vi "Recursive Find Config File.vi"(8 "error in":errorcluster, 10 "Path":path, 11 "Configuration in":refnum<class "Configuration.lvclass">) -> (0 "error out":errorcluster, 2 "File Path":path, 3 "Configuration out":refnum<class "Configuration.lvclass">)   [LabVIEW 2018, in "Configuration.lvlib" / "Configuration.lvclass"]
doc: "This is a recursive file searcher. \n\nIt starts at an input path, moves up one directory and searches for config.ini\n\nTypical practice is to pass in the application path which will root the search in the projoct folders looking in higher level folders."
uses:
  Configuration.lvclass
  Configuration.lvclass/Configuration.ctl
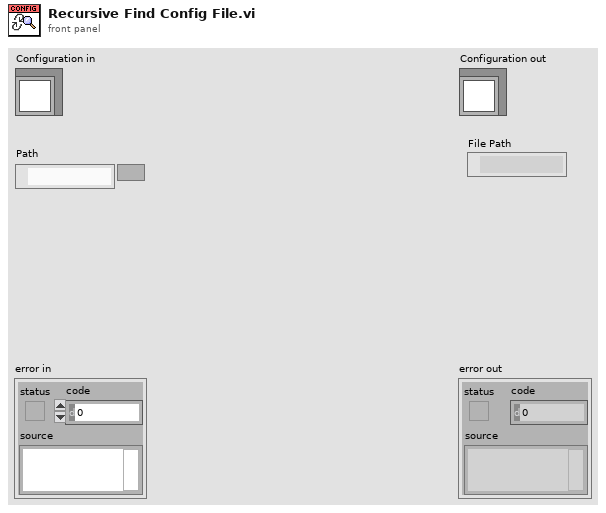
[diagram p1: front panel]
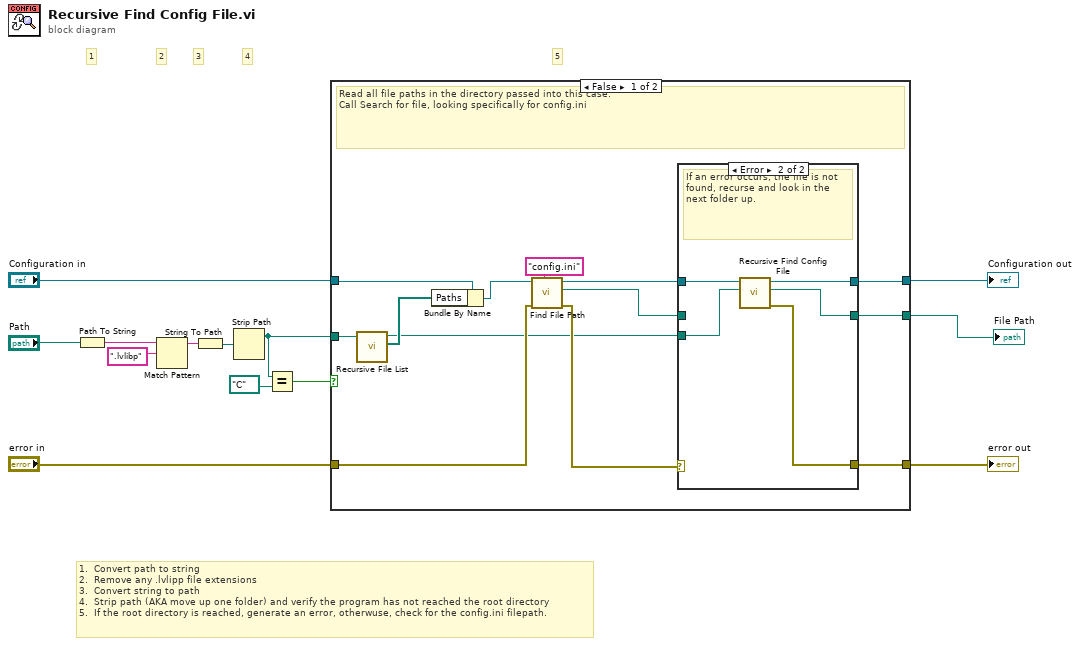
[diagram p0: block diagram]
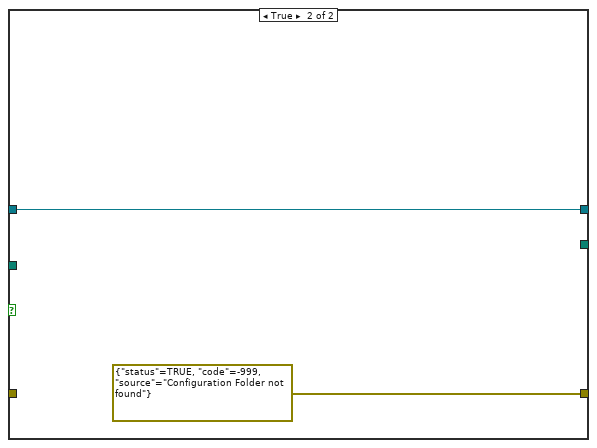
[diagram p3: hidden frame]
diagram:
  # "1.  Convert path to string\n2.  Remove any .lvlipp file extensions\n3.  Convert string to path\n4.  Strip path (AKA move up one folder) and verify the program has not reached the root directory\n5.  If the root directory is reached, generate an error, otherwuse, check for the config.ini filepath."
  # "5"
  # "4"
  # "3"
  # "2"
  # "1"
  n1 = Path To String(path="Path") -> (string=w12:string)
  n2 = Match Pattern(string=w12, regular expression=".lvlibp") -> (before substring=w10:string)  [unwired: 1 in, 3 out]
  n3 = String To Path(string=w10) -> (path=w9:path)
  n4 = Strip Path(path=w9) -> (stripped path=w6:path)  [unwired: 1 out]
  n5 = Equal?(x=w6, y=path "C:/" ("stripped path")) -> (x = y?=w7:bool)
  n6 = case shown="False" w7 {
    tunnel: w6 -> [w23 _]
    tunnel: "Configuration in" -> [w26 w36]
    tunnel: [w16 w36] -> w4
    tunnel: "error in" -> [w24 _]
    tunnel: [w15 errorcluster {"status"=TRUE, "code"=-999, "source"="Configuration Folder not found"} ("error in")] -> w2
    tunnel: [w18 _] -> w1
    frame False {
      # "Read all file paths in the directory passed into this case.\nCall Search for file, looking specifically for config.ini"
      n7 = call <vilib>:"Recursive File List.vi"("Folder Path"=w23) -> ("All Files in Dir"=w21:path[], "dup Folder Path"=w14:path)  [unwired: 6 in, 3 out]
      n8 = Bundle By Name(cluster=w26, "Paths"=w21) -> (w22:refnum<class "Configuration.lvclass">)
      n9 = call "Find File Path.vi"("error in"=w24, "Filename"="config.ini", "Configuration in"=w22) -> ("error out"=w20:errorcluster, "File Path"=w19:path, "Configuration out"=w17:refnum<class "Configuration.lvclass">)  [unwired: 6 in]
      n10 = case shown="Error" w20 {
        selector: w20 -> [w27 _]
        tunnel: w19 -> [w29 _]
        tunnel: [w29 w31] -> w18
        tunnel: w17 -> [w28 w34]
        tunnel: [w28 w33] -> w16
        tunnel: [w27 w32] -> w15
        tunnel: w14 -> [_ w30]
        frame No Error {
          # "If no error is generated, the file has been found, return the file path."
        }
        frame Error {
          # "If an error occurs, the file is not found, recurse and look in the next folder up."
          n11 = call "Recursive Find Config File.vi"("Path"=w30, "Configuration in"=w34) -> ("error out"=w32:errorcluster, "File Path"=w31:path, "Configuration out"=w33:refnum<class "Configuration.lvclass">)  [unwired: 7 in]
        }
      }
    }
    frame True {
    }
  }
  "error out" <- w2
  "Configuration out" <- w4
  "File Path" <- w1
